vi "unflatten memory.vi"(8 "error in":errorcluster, 10 "binary repo":string, 11 "CEF_HierarchyRepo in":refnum<class "CEF_HierarchyRepo.lvclass">) -> (0 "error out":errorcluster, 3 "CEF_HierarchyRepo out":refnum<class "CEF_HierarchyRepo.lvclass">)   [LabVIEW 2025, in "CEF.lvlib" / "CEF_HierarchyRepo.lvclass"]
doc: "Copyright 2017 National Instruments Corporation\n\nLicensed under the Apache License, Version 2.0 (the \"License\"); you may not use this file except in compliance with the License. You may obtain a copy of the License at http://www.apache.org/licenses/LICENSE-2.0\nUnless required by applicable law or agreed to in writing, software distributed under the License is distributed on an \"AS IS\" BASIS, WITHOUT WARRANTIES OR CONDITIONS OF ANY KIND, either express or implied. See the License for the specific language governing permissions and limitations under the License."
uses:
  CEF_HierarchyRepo.lvclass
  memory hierarchy.ctl
  full hierarchy.ctl
  tree serializer/hierarchy element.ctl
  serializable configuration/CEF_serializable configuration.lvclass
  CEF_HierarchyRepo.lvclass/CEF_HierarchyRepo.ctl
  CEF.lvlib
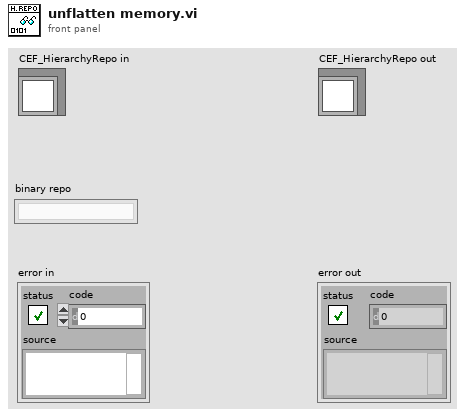
[diagram p1: front panel]
types:
  T1 = typedef "CEF.lvlib/CEF_HierarchyRepo.lvclass/memory hierarchy.ctl" = cluster{"hierarchy structure":T2, "instance data":refnum<class "CEF_serializable configuration.lvclass">[]}
  T2 = typedef "CEF.lvlib/CEF_HierarchyRepo.lvclass/full hierarchy.ctl" = cluster{"root":string, "hierarchy":T3[]}
  T3 = typedef "CEF.lvlib/hierarchy element.ctl" = cluster{"current node":string, "children":string[]}
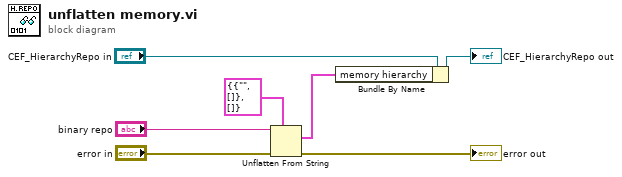
[diagram p0: block diagram]
diagram:
  n1 = Unflatten From String(type=T1 {"hierarchy structure"={"root"="", "hierarchy"=[]}, "instance data"=[]} ("memory hierarchy"), binary string="binary repo", error in (no error)="error in") -> (value=w1:T1, error out=→"error out":errorcluster)  [unwired: 2 in, 1 out]
  n2 = Bundle By Name(cluster="CEF_HierarchyRepo in", "memory hierarchy"=w1) -> (→"CEF_HierarchyRepo out":refnum<class "CEF_HierarchyRepo.lvclass">)
